vi "PCO_Description.vi"() -> (0 "PCO_Description":T2 {"wSensorTypeDESC" format="%x"; "wSensorSubTypeDESC" format="%x"; "wColorPatternDESC" format="%x"; "wPatternTypeDESC" format="%x"; "dwGeneralCapsDESC2" format="%x"; "dwGeneralCapsDESC3" format="%x"; "dwGeneralCapsDESC4" format="%x"}, 1 "PCO_Description_Raw":T1, 2 "Length":u16, 3 "Raw_Length":u16)   [LabVIEW 2020, in "SDK.lvlib" / "Structures.lvlib"]
doc: "Use this template to build a VI to use as a subVI."
uses:
  Structures.lvlib
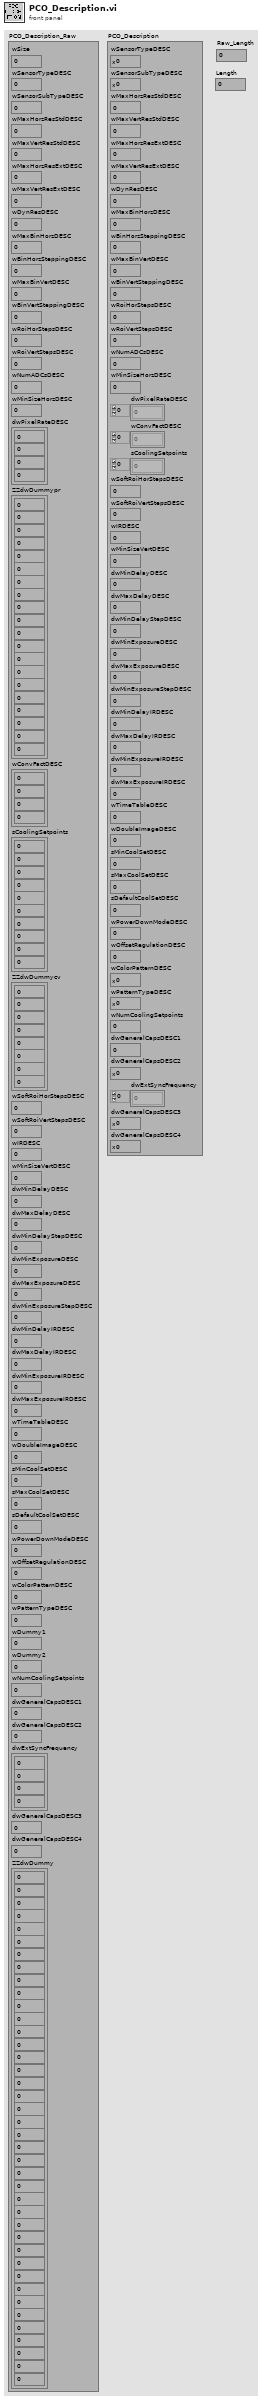
[diagram p1: front panel]
types:
  T1 = cluster{"wSize":u16, "wSensorTypeDESC":u16, "wSensorSubTypeDESC":u16, "wMaxHorzResStdDESC":u16, "wMaxVertResStdDESC":u16, "wMaxHorzResExtDESC":u16, "wMaxVertResExtDESC":u16, "wDynResDESC":u16, "wMaxBinHorzDESC":u16, "wBinHorzSteppingDESC":u16, "wMaxBinVertDESC":u16, "wBinVertSteppingDESC":u16, "wRoiHorStepsDESC":u16, "wRoiVertStepsDESC":u16, "wNumADCsDESC":u16, "wMinSizeHorzDESC":u16, "dwPixelRateDESC":cluster{u32, u32, u32, u32}, "ZZdwDummypr":cluster{u32, u32, u32, u32, u32, u32, u32, u32, u32, u32, u32, u32, u32, u32, u32, u32, u32, u32, u32, u32}, "wConvFactDESC":cluster{u16, u16, u16, u16}, "sCoolingSetpoints":cluster{i16, i16, i16, i16, i16, i16, i16, i16, i16, i16}, "ZZdwDummycv":cluster{u16, u16, u16, u16, u16, u16, u16, u16}, "wSoftRoiHorStepsDESC":u16, "wSoftRoiVertStepsDESC":u16, "wIRDESC":u16, "wMinSizeVertDESC":u16, "dwMinDelayDESC":u32, "dwMaxDelayDESC":u32, "dwMinDelayStepDESC":u32, "dwMinExposureDESC":u32, "dwMaxExposureDESC":u32, "dwMinExposureStepDESC":u32, "dwMinDelayIRDESC":u32, "dwMaxDelayIRDESC":u32, "dwMinExposureIRDESC":u32, "dwMaxExposureIRDESC":u32, "wTimeTableDESC":u16, "wDoubleImageDESC":u16, "sMinCoolSetDESC":i16, "sMaxCoolSetDESC":i16, "sDefaultCoolSetDESC":i16, "wPowerDownModeDESC":u16, "wOffsetRegulationDESC":u16, "wColorPatternDESC":u16, "wPatternTypeDESC":u16, "wDummy1":u16, "wDummy2":u16, "wNumCoolingSetpoints":u16, "dwGeneralCapsDESC1":u32, "dwGeneralCapsDESC2":u32, "dwExtSyncFrequency":cluster{u32, u32, u32, u32}, "dwGeneralCapsDESC3":u32, "dwGeneralCapsDESC4":u32, "ZZdwDummy":cluster{u32, u32, u32, u32, u32, u32, u32, u32, u32, u32, u32, u32, u32, u32, u32, u32, u32, u32, u32, u32, u32, u32, u32, u32, u32, u32, u32, u32, u32, u32, u32, u32, u32, u32, u32, u32, u32, u32, u32, u32}}
  T2 = cluster{"wSensorTypeDESC":u16, "wSensorSubTypeDESC":u16, "wMaxHorzResStdDESC":u16, "wMaxVertResStdDESC":u16, "wMaxHorzResExtDESC":u16, "wMaxVertResExtDESC":u16, "wDynResDESC":u16, "wMaxBinHorzDESC":u16, "wBinHorzSteppingDESC":u16, "wMaxBinVertDESC":u16, "wBinVertSteppingDESC":u16, "wRoiHorStepsDESC":u16, "wRoiVertStepsDESC":u16, "wNumADCsDESC":u16, "wMinSizeHorzDESC":u16, "dwPixelRateDESC":u32[], "wConvFactDESC":u16[], "sCoolingSetpoints":i16[], "wSoftRoiHorStepsDESC":u16, "wSoftRoiVertStepsDESC":u16, "wIRDESC":u16, "wMinSizeVertDESC":u16, "dwMinDelayDESC":u32, "dwMaxDelayDESC":u32, "dwMinDelayStepDESC":u32, "dwMinExposureDESC":u32, "dwMaxExposureDESC":u32, "dwMinExposureStepDESC":u32, "dwMinDelayIRDESC":u32, "dwMaxDelayIRDESC":u32, "dwMinExposureIRDESC":u32, "dwMaxExposureIRDESC":u32, "wTimeTableDESC":u16, "wDoubleImageDESC":u16, "sMinCoolSetDESC":i16, "sMaxCoolSetDESC":i16, "sDefaultCoolSetDESC":i16, "wPowerDownModeDESC":u16, "wOffsetRegulationDESC":u16, "wColorPatternDESC":u16, "wPatternTypeDESC":u16, "wNumCoolingSetpoints":u16, "dwGeneralCapsDESC1":u32, "dwGeneralCapsDESC2":u32, "dwExtSyncFrequency":u32[], "dwGeneralCapsDESC3":u32, "dwGeneralCapsDESC4":u32}
  T3 = cluster{u32, u32, u32, u32, u32, u32, u32, u32, u32, u32, u32, u32, u32, u32, u32, u32, u32, u32, u32, u32, u32, u32, u32, u32, u32, u32, u32, u32, u32, u32, u32, u32, u32, u32, u32, u32, u32, u32, u32, u32}
  T4 = cluster{i16, i16, i16, i16, i16, i16, i16, i16, i16, i16}
  T5 = cluster{u32, u32, u32, u32, u32, u32, u32, u32, u32, u32, u32, u32, u32, u32, u32, u32, u32, u32, u32, u32}
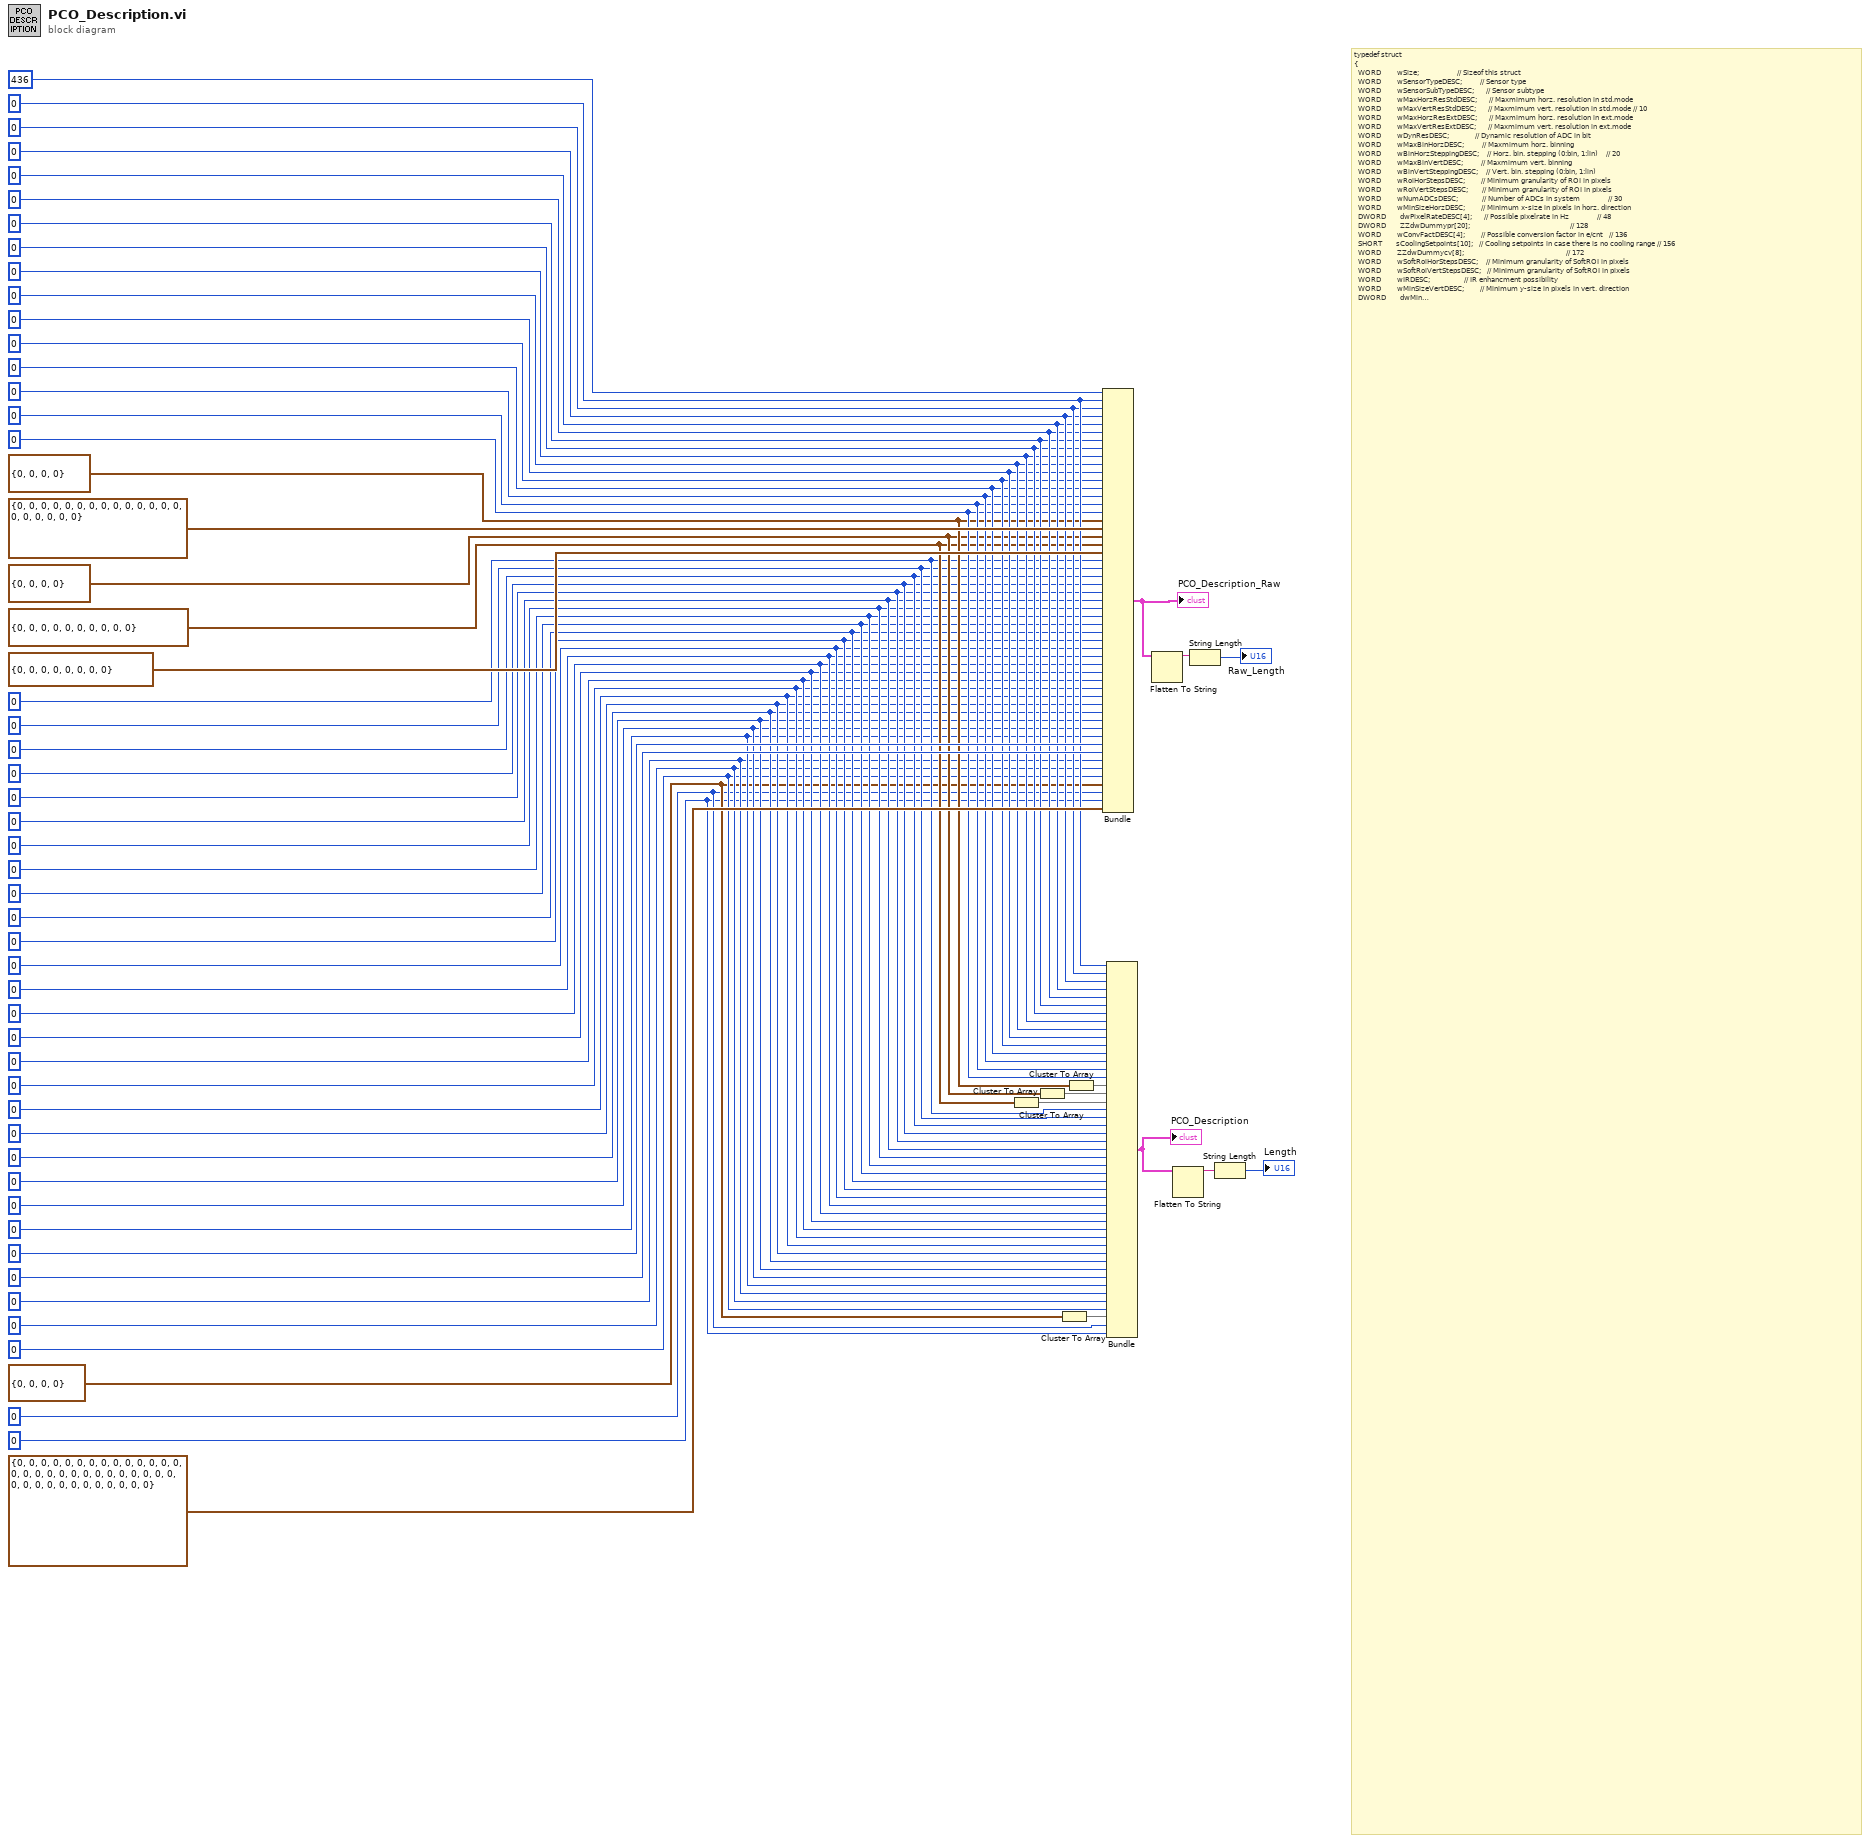
[diagram p0: block diagram]
diagram:
  w2 = u32 0 ("dwGeneralCapsDESC4")
  w3 = u32 0 ("dwGeneralCapsDESC3")
  w5 = cluster{u32, u32, u32, u32} {0, 0, 0, 0} ("dwExtSyncFrequency")
  w6 = u32 0 ("dwGeneralCapsDESC2")
  w7 = u32 0 ("dwGeneralCapsDESC1")
  w8 = u16 0 ("wNumCoolingSetpoints")
  w9 = u16 0 ("wPatternTypeDESC")
  w10 = u16 0 ("wColorPatternDESC")
  w11 = u16 0 ("wOffsetRegulationDESC")
  w12 = u16 0 ("wPowerDownModeDESC")
  w13 = i16 0 ("sDefaultCoolSetDESC")
  w14 = i16 0 ("sMaxCoolSetDESC")
  w15 = i16 0 ("sMinCoolSetDESC")
  w16 = u16 0 ("wDoubleImageDESC")
  w17 = u16 0 ("wTimeTableDESC")
  w18 = u32 0 ("dwMaxExposureIRDESC")
  w19 = u32 0 ("dwMinExposureIRDESC")
  w20 = u32 0 ("dwMaxDelayIRDESC")
  w21 = u32 0 ("dwMinDelayIRDESC")
  w22 = u32 0 ("dwMinExposureStepDESC")
  w23 = u32 0 ("dwMaxExposureDESC")
  w24 = u32 0 ("dwMinExposureDESC")
  w25 = u32 0 ("dwMinDelayStepDESC")
  w26 = u32 0 ("dwMaxDelayDESC")
  w27 = u32 0 ("dwMinDelayDESC")
  w28 = u16 0 ("wMinSizeVertDESC")
  w29 = u16 0 ("wIRDESC")
  w30 = u16 0 ("wSoftRoiVertStepsDESC")
  w31 = u16 0 ("wSoftRoiHorStepsDESC")
  w33 = T4 {0, 0, 0, 0, 0, 0, 0, 0, 0, 0} ("sCoolingSetpoints")
  w35 = cluster{u16, u16, u16, u16} {0, 0, 0, 0} ("wConvFactDESC")
  w36 = cluster{u32, u32, u32, u32} {0, 0, 0, 0} ("dwPixelRateDESC")
  w38 = u16 0 ("wMinSizeHorzDESC")
  w39 = u16 0 ("wNumADCsDESC")
  w40 = u16 0 ("wRoiVertStepsDESC")
  w41 = u16 0 ("wRoiHorStepsDESC")
  w42 = u16 0 ("wBinVertSteppingDESC")
  w43 = u16 0 ("wMaxBinVertDESC")
  w44 = u16 0 ("wBinHorzSteppingDESC")
  w45 = u16 0 ("wMaxBinHorzDESC")
  w46 = u16 0 ("wDynResDESC")
  w47 = u16 0 ("wMaxVertResExtDESC")
  w48 = u16 0 ("wMaxHorzResExtDESC")
  w49 = u16 0 ("wMaxVertResStdDESC")
  w50 = u16 0 ("wMaxHorzResStdDESC")
  w51 = u16 0 ("wSensorSubTypeDESC")
  w52 = u16 0 ("wSensorTypeDESC")
  # "typedef struct\n{\n  WORD        wSize;                   // Sizeof this struct\n  WORD        wSensorTypeDESC;         // Sensor type\n  WORD        wSensorSubTypeDESC;      // Sensor subtype\n  WORD        wMaxHorzResStdDESC;      // Maxmimum horz. resolution in std.mode\n  WORD        wMaxVertResStdDESC;      // Maxmimum vert. resolution in std.mode // 10\n  WORD        wMaxHorzResExtDESC;      // Maxmimum horz. resolution in ext.mode\n  WORD        wMaxVertResExtDESC;      // Maxmimum vert. resolution in ext.mode\n  WORD        wDynResDESC;             // Dynamic resolution of ADC in bit\n  WORD        wMaxBinHorzDESC;         // Maxmimum horz. binning\n  WORD        wBinHorzSteppingDESC;    // Horz. bin. stepping (0:bin, 1:lin)    // 20\n  WORD        wMaxBinVertDESC;         // Maxmimum vert. binning\n  WORD        wBinVertSteppingDESC;    // Vert. bin. stepping (0:bin, 1:lin)\n  WORD        wRoiHorStepsDESC;        // Minimum granularity of ROI in pixels\n  WORD        wRoiVertStepsDESC;       // Minimum granularity of ROI in pixels\n  WORD        wNumADCsDESC;            // Number of ADCs in system              // 30\n  WORD        wMinSizeHorzDESC;        // Minimum x-size in pixels in horz. direction\n  DWORD       dwPixelRateDESC[4];      // Possible pixelrate in Hz              // 48\n  DWORD       ZZdwDummypr[20];                                                  // 128\n  WORD        wConvFactDESC[4];        // Possible conversion factor in e/cnt   // 136\n  SHORT       sCoolingSetpoints[10];   // Cooling setpoints in case there is no cooling range // 156\n  WORD        ZZdwDummycv[8];                                                   // 172\n  WORD        wSoftRoiHorStepsDESC;    // Minimum granularity of SoftROI in pixels\n  WORD        wSoftRoiVertStepsDESC;   // Minimum granularity of SoftROI in pixels\n  WORD        wIRDESC;                 // IR enhancment possibility\n  WORD        wMinSizeVertDESC;        // Minimum y-size in pixels in vert. direction\n  DWORD       dwMinDelayDESC;          // Minimum delay time in ns\n  DWORD       dwMaxDelayDESC;          // Maximum delay time in ms\n  DWORD       dwMinDelayStepDESC;      // Minimum stepping of delay time in ns  // 192\n  DWORD       dwMinExposureDESC;       // Minimum exposure time in ns\n  DWORD       dwMaxExposureDESC;       // Maximum exposure time in ms           // 200\n  DWORD       dwMinExposureStepDESC;   // Minimum stepping of exposure time in ns\n  DWORD       dwMinDelayIRDESC;        // Minimum delay time in ns\n  DWORD       dwMaxDelayIRDESC;        // Maximum delay time in ms              // 212\n  DWORD       dwMinExposureIRDESC;     // Minimum exposure time in ns\n  DWORD       dwMaxExposureIRDESC;     // Maximum exposure time in ms           // 220\n  WORD        wTimeTableDESC;          // Timetable for exp/del possibility\n  WORD        wDoubleImageDESC;        // Double image mode possibility\n  SHORT       sMinCoolSetDESC;         // Minimum value for cooling\n  SHORT       sMaxCoolSetDESC;         // Maximum value for cooling\n  SHORT       sDefaultCoolSetDESC;     // Default value for cooling             // 230\n  WORD        wPowerDownModeDESC;      // Power down mode possibility\n  WORD        wOffsetRegulationDESC;   // Offset regulation possibility\n  WORD        wColorPatternDESC;       // Color pattern of color chip\n                                       // four nibbles (0,1,2,3) in word \n                                       //  ----------------- \n                                       //  | 3 | 2 | 1 | 0 |\n                                       //  ----------------- \n                                       //   \n                                       // describe row,column  2,2 2,1 1,2 1,1\n                                       // \n                                       //   column1 column2\n                                       //  ----------------- \n                                       //  |       |       |\n                                       //  |   0   |   1   |   row1\n                                       //  |       |       |\n                                       //  -----------------\n                                       //  |       |       |\n                                       //  |   2   |   3   |   row2\n                                       //  |       |       |\n                                       //  -----------------\n                                       // \n  WORD        wPatternTypeDESC;        // Pattern type of color chip\n                                       // 1: Bayer pattern RGB\n  WORD        wDummy1;                 // former DSNU correction mode             // 240\n  WORD        wDummy2;                 // \n  WORD        wNumCoolingSetpoints;    //\n  DWORD       dwGeneralCapsDESC1;      // General capabilities:\n                                       // Bit 0: Noisefilter available\n                                       // Bit 1: Hotpixelfilter available\n                                       // Bit 2: Hotpixel works only with noisefilter\n                                       // Bit 3: Timestamp ASCII only available (Timestamp mode 3 enabled)\n\n                                       // Bit 4: Dataformat 2x12\n                                       // Bit 5: Record Stop Event available\n                                       // Bit 6: Hot Pixel correction\n                                       // Bit 7: Ext.Exp.Ctrl. not available\n\n                                       // Bit 8: Timestamp not available\n                                       // Bit 9: Acquire mode not available\n                                       // Bit10: Dataformat 4x16\n                                       // Bit11: Dataformat 5x16\n\n                                       // Bit12: Camera has no internal recorder memory\n                                       // Bit13: Camera can be set to fast timing mode (PIV)\n                                       // Bit14: Camera can produce metadata\n                                       // Bit15: Camera allows Set/GetFrameRate cmd\n\n                                       // Bit16: Camera has Correlated Double Image Mode\n                                       // Bit17: Camera has CCM\n                                       // Bit18: Camera can be synched externally\n                                       // Bit19: Global shutter setting not available\n\n                                       // Bit20: Camera supports global reset rolling readout\n                                       // Bit21: Camera supports extended acquire command\n                                       // Bit22: Camera supports fan control command\n                                       // Bit23: Camera vert.ROI must be symmetrical to horizontal axis\n\n                                       // Bit24: Camera horz.ROI must be symmetrical to vertical axis\n                                       // Bit25: Camera has cooling setpoints instead of cooling range\n\n                                       // Bit26: \n                                       // Bit27: reserved for future use\n                                       \n                                       // Bit28: reserved for future desc.// Bit29:  reserved for future desc.\n\n                                       // Bit 30: HW_IO_SIGNAL_DESCRIPTOR available\n                                       // Bit 31: Enhanced descriptor available\n\n  DWORD       dwGeneralCapsDESC2;      // General capabilities 2                  // 252\n                                       // Bit 0 ... 29: reserved for future use\n                                       // Bit 30: used internally (sc2_defs_intern.h)\n                                       // Bit 31: used internally (sc2_defs_intern.h)\n  DWORD       dwExtSyncFrequency[4];   // lists four frequencies for external sync feature\n  DWORD       dwGeneralCapsDESC3;      // general capabilites descr. 3 \n  DWORD       dwGeneralCapsDESC4;      // general capabilites descr. 4            // 276\n  DWORD       ZZdwDummy[40];                                                      // 436\n} PCO_Description;"
  n1 = Cluster To Array(cluster=w33) -> (array=w32:i16[])
  n2 = Cluster To Array(cluster=w35) -> (array=w34:u16[])
  n3 = Cluster To Array(cluster=w5) -> (array=w4:u32[])
  n4 = Cluster To Array(cluster=w36) -> (array=w37:u32[])
  n5 = Bundle("wSize"=u16 436, "wSensorTypeDESC"=w52, "wSensorSubTypeDESC"=w51, "wMaxHorzResStdDESC"=w50, "wMaxVertResStdDESC"=w49, "wMaxHorzResExtDESC"=w48, "wMaxVertResExtDESC"=w47, "wDynResDESC"=w46, "wMaxBinHorzDESC"=w45, "wBinHorzSteppingDESC"=w44, "wMaxBinVertDESC"=w43, "wBinVertSteppingDESC"=w42, "wRoiHorStepsDESC"=w41, "wRoiVertStepsDESC"=w40, "wNumADCsDESC"=w39, "wMinSizeHorzDESC"=w38, "dwPixelRateDESC"=w36, "ZZdwDummypr"=T5 {0, 0, 0, 0, 0, 0, 0, 0, 0, 0, 0, 0, 0, 0, 0, 0, 0, 0, 0, 0}, "wConvFactDESC"=w35, "sCoolingSetpoints"=w33, "ZZdwDummycv"=cluster{u16, u16, u16, u16, u16, u16, u16, u16} {0, 0, 0, 0, 0, 0, 0, 0}, "wSoftRoiHorStepsDESC"=w31, "wSoftRoiVertStepsDESC"=w30, "wIRDESC"=w29, "wMinSizeVertDESC"=w28, "dwMinDelayDESC"=w27, "dwMaxDelayDESC"=w26, "dwMinDelayStepDESC"=w25, "dwMinExposureDESC"=w24, "dwMaxExposureDESC"=w23, "dwMinExposureStepDESC"=w22, "dwMinDelayIRDESC"=w21, "dwMaxDelayIRDESC"=w20, "dwMinExposureIRDESC"=w19, "dwMaxExposureIRDESC"=w18, "wTimeTableDESC"=w17, "wDoubleImageDESC"=w16, "sMinCoolSetDESC"=w15, "sMaxCoolSetDESC"=w14, "sDefaultCoolSetDESC"=w13, "wPowerDownModeDESC"=w12, "wOffsetRegulationDESC"=w11, "wColorPatternDESC"=w10, "wPatternTypeDESC"=w9, "wDummy1"=u16 0, "wDummy2"=u16 0, "wNumCoolingSetpoints"=w8, "dwGeneralCapsDESC1"=w7, "dwGeneralCapsDESC2"=w6, "dwExtSyncFrequency"=w5, "dwGeneralCapsDESC3"=w3, "dwGeneralCapsDESC4"=w2, "ZZdwDummy"=T3 {0, 0, 0, 0, 0, 0, 0, 0, 0, 0, 0, 0, 0, 0, 0, 0, 0, 0, 0, 0, 0, 0, 0, 0, 0, 0, 0, 0, 0, 0, 0, 0, 0, 0, 0, 0, 0, 0, 0, 0}) -> (w1:T1)  [unwired: 1 in]
  "PCO_Description_Raw" <- w1
  n6 = Bundle("wSensorTypeDESC"=w52, "wSensorSubTypeDESC"=w51, "wMaxHorzResStdDESC"=w50, "wMaxVertResStdDESC"=w49, "wMaxHorzResExtDESC"=w48, "wMaxVertResExtDESC"=w47, "wDynResDESC"=w46, "wMaxBinHorzDESC"=w45, "wBinHorzSteppingDESC"=w44, "wMaxBinVertDESC"=w43, "wBinVertSteppingDESC"=w42, "wRoiHorStepsDESC"=w41, "wRoiVertStepsDESC"=w40, "wNumADCsDESC"=w39, "wMinSizeHorzDESC"=w38, "dwPixelRateDESC"=w37, "wConvFactDESC"=w34, "sCoolingSetpoints"=w32, "wSoftRoiHorStepsDESC"=w31, "wSoftRoiVertStepsDESC"=w30, "wIRDESC"=w29, "wMinSizeVertDESC"=w28, "dwMinDelayDESC"=w27, "dwMaxDelayDESC"=w26, "dwMinDelayStepDESC"=w25, "dwMinExposureDESC"=w24, "dwMaxExposureDESC"=w23, "dwMinExposureStepDESC"=w22, "dwMinDelayIRDESC"=w21, "dwMaxDelayIRDESC"=w20, "dwMinExposureIRDESC"=w19, "dwMaxExposureIRDESC"=w18, "wTimeTableDESC"=w17, "wDoubleImageDESC"=w16, "sMinCoolSetDESC"=w15, "sMaxCoolSetDESC"=w14, "sDefaultCoolSetDESC"=w13, "wPowerDownModeDESC"=w12, "wOffsetRegulationDESC"=w11, "wColorPatternDESC"=w10, "wPatternTypeDESC"=w9, "wNumCoolingSetpoints"=w8, "dwGeneralCapsDESC1"=w7, "dwGeneralCapsDESC2"=w6, "dwExtSyncFrequency"=w4, "dwGeneralCapsDESC3"=w3, "dwGeneralCapsDESC4"=w2) -> (w63:T2)  [unwired: 1 in]
  "PCO_Description" <- w63
  n7 = Flatten To String(anything=w1) -> (data string=w61:string)  [unwired: 3 in, 2 out]
  n8 = Flatten To String(anything=w63) -> (data string=w62:string)  [unwired: 3 in, 2 out]
  n9 = String Length(string=w61) -> (length=→"Raw_Length":i32)
  n10 = String Length(string=w62) -> (length=→"Length":i32)
